vi "Set Configuration.vi"(8 "error in (no error)":errorcluster, 11 "EST Input in":refnum<class "EST Input.lvclass">) -> (0 "error out":errorcluster, 3 "EST Input out":refnum<class "EST Input.lvclass">)   [LabVIEW 2015, in "EST Input.lvclass"]
uses:
  EST Input.lvclass
  IO Class/Classification.ctl
  Input Signal/Input Signal.lvclass
  IO Class/IO Class.lvclass
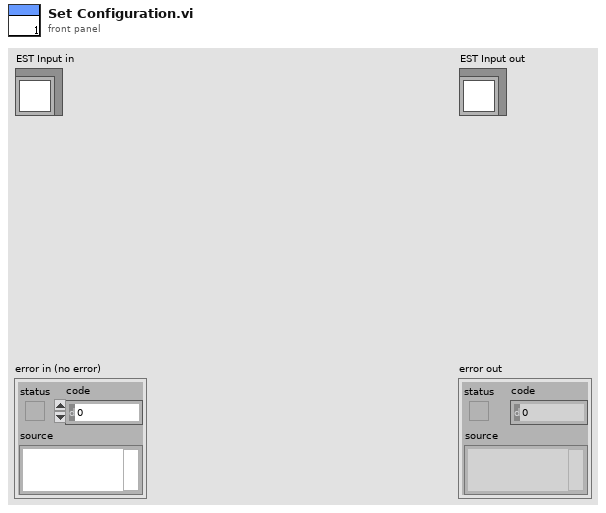
[diagram p1: front panel]
types:
  T1 = typedef "IO Class.lvclass/Classification.ctl" = cluster{"Classification":string}
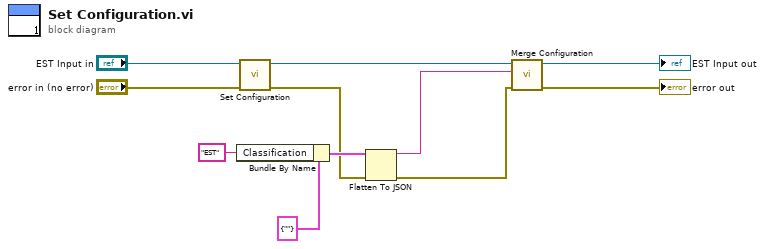
[diagram p0: block diagram]
diagram:
  n1 = Bundle By Name(cluster=T1 {"Classification"=""} ("Classification"), "Classification"="EST" ("Type")) -> (w10:T1)
  n2 = call-parent "Set Configuration.vi"("error in (no error)"="error in (no error)", "Input Signal in"="EST Input in") -> ("error out"=w9:errorcluster, "Input Signal out"=w7:refnum<class "EST Input.lvclass">)  [unwired: 8 in]
  n3 = Flatten To JSON(anything=w10, error in (no error)=w9) -> (JSON string=w6:string, 11:w8:errorcluster)  [unwired: 1 in]
  n4 = call "Merge Configuration.vi"("error in (no error)"=w8, "Additional Configuration"=w6, "IO Class in"=w7) -> ("error out"=→"error out":errorcluster, "IO Class out"=→"EST Input out":refnum<class "EST Input.lvclass">)  [unwired: 7 in]
